vi "LuaVIEW Get Function Info.vi"(0 "function VI name (use path)":string, 7 "function VI path":path, 11 "error in (no error)":errorcluster) -> (8 "function info":T1, 15 "error out":errorcluster)   [LabVIEW 2012]
doc: "Extract the function info (excluding docstring and synopsis) from a LuaVIEW function VI. If the VI of that name is already in memory a partial path can be used and a different path might be returned than the one supplied."
uses:
  typedefs/clusters/LuaVIEW Function Info.ctl
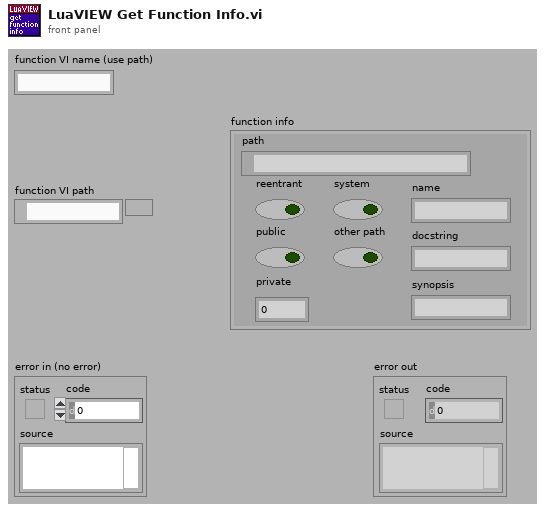
[diagram p1: front panel]
types:
  T1 = typedef "LuaVIEW Function Info.ctl" = cluster{"path":path, "reentrant":bool, "public":bool, "private":i32, "system":bool, "other path":bool, "name":string, "docstring":string, "synopsis":string}
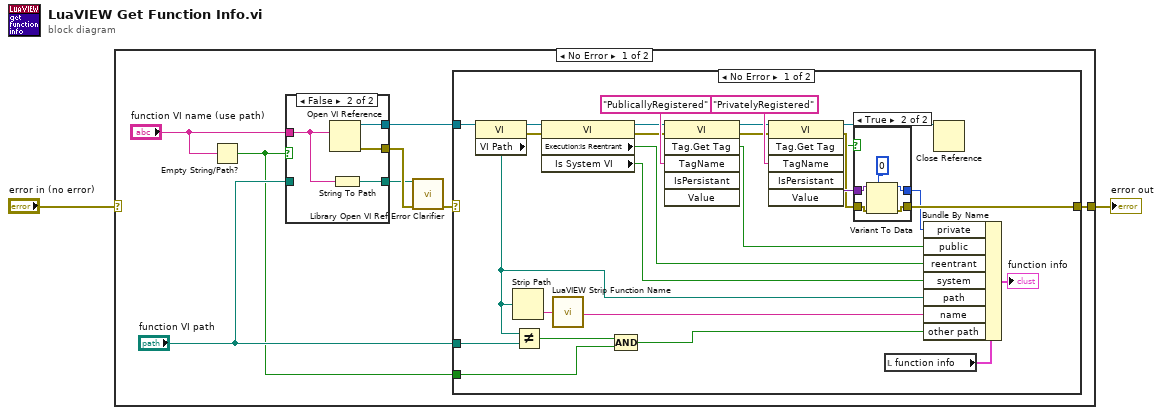
[diagram p0: block diagram]
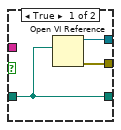
[diagram p2: hidden frame]
diagram:
  n1 = case shown="No Error" "error in (no error)" {
    selector: "error in (no error)" -> [_ w52]
    tunnel: [w7 w52] -> w1
    frame No Error {
      n2 = Empty String/Path?(string/path="function VI name (use path)") -> (empty?=w3:bool)
      n3 = case shown="False" w3 {
        tunnel: [w13 w17] -> w10
        tunnel: [w12 w16] -> w9
        tunnel: "function VI path" -> [w11 _]
        tunnel: [w11 w14] -> w5
        tunnel: "function VI name (use path)" -> [_ w15]
        frame True {
          n4 = Open VI Reference(vi path=w11) -> (vi reference=w12:refnum<vi>, error out=w13:errorcluster)  [unwired: 5 in]
        }
        frame False {
          n5 = Open VI Reference(vi path=w15) -> (vi reference=w16:refnum<vi>, error out=w17:errorcluster)  [unwired: 5 in]
          n6 = String To Path(string=w15) -> (path=w14:path)
        }
      }
      n7 = call "Library Open VI Ref Error Clarifier.vi"("VI path"=w5, "called VI error (no error)"=w10) -> ("error out"=w8:errorcluster)  [unwired: 13 in]
      n8 = case shown="No Error" w8 {
        selector: w8 -> [_ w51]
        tunnel: w9 -> [w42 _]
        tunnel: [w31 w51] -> w7
        tunnel: "function VI path" -> [w29 _]
        tunnel: w3 -> [w18 _]
        frame No Error {
          n9 = property class="VI"(reference=w42) -> (reference out=w28:refnum<vi>, error out=w27:errorcluster, "VI Path"=w19:path)  [unwired: 1 in]
          n10 = Strip Path(path=w19) -> (name=w35:string)  [unwired: 1 out]
          n11 = Not Equal?(x=w19, y=w29) -> (x != y?=w21:bool)
          n12 = property class="VI"(reference=w28, error in=w27) -> (reference out=w26:refnum<vi>, error out=w25:errorcluster, "Execution:Is Reentrant"=w24:bool, "Is System VI"=w23:bool)
          n13 = call "LuaVIEW Strip Function Name.vi"("function VI name"=w35) -> ("Lua function name"=w22:string)  [unwired: 14 in]
          n14 = Compound Arithmetic op=AND(w21, w18) -> (w20:bool)
          n15 = invoke class="VI" method="Tag.Get Tag"(reference=w26, error in=w25, "TagName"="PublicallyRegistered") -> (reference out=w39:refnum<vi>, error out=w38:errorcluster, "GetTag"=w36:bool)  [unwired: 3 in, 3 out]
          n16 = invoke class="VI" method="Tag.Get Tag"(reference=w39, error in=w38, "TagName"="PrivatelyRegistered") -> (reference out=w37:refnum<vi>, error out=w33:errorcluster, "GetTag"=w32:bool, "Value"=w34:variant)  [unwired: 3 in, 2 out]
          n17 = case shown="True" w32 {
            tunnel: w34 -> [_ w50]
            tunnel: w33 -> [w45 w49]
            tunnel: [w45 w47] -> w31
            tunnel: [_ w46] -> w30
            frame False {
            }
            frame True {
              n18 = Variant To Data(error in=w49, type=0, Variant=w50) -> (data=w46:i32, error out=w47:errorcluster)
            }
          }
          n19 = local read "function info"() -> (w44:T1)
          n20 = Bundle By Name(cluster=w44, "private"=w30, "public"=w36, "reentrant"=w24, "system"=w23, "path"=w19, "name"=w22, "other path"=w20) -> (→"function info":T1)
          n21 = Close Reference(reference=w37) -> ()  [unwired: 1 in, 1 out]
        }
        frame Error {
        }
      }
    }
    frame Error {
    }
  }
  "error out" <- w1
